vi "initialize_oscilloscope_multiple_waveforms.vi"(0 "Range (0.001 S)":dbl=1.0 format="%#_13g", 1 "error in (no error)":errorcluster) -> (2 "VISA resource name out":refnum<visa-resource-name>, 3 "channels":i32[](array[numeric]), 4 "error out":errorcluster)   [LabVIEW 2016]
doc: "This example shows how to configure multiple channels and acquire waveforms from multiple channels."
uses:
  <instrlib>/Agilent 2000 3000 X-Series/Agilent 2000 3000 X-Series.lvlib
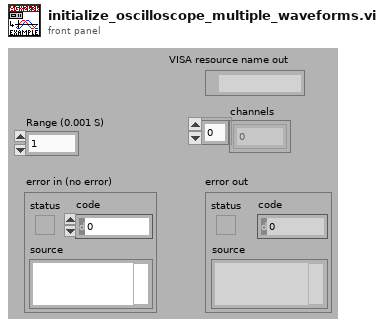
[diagram p1: front panel]
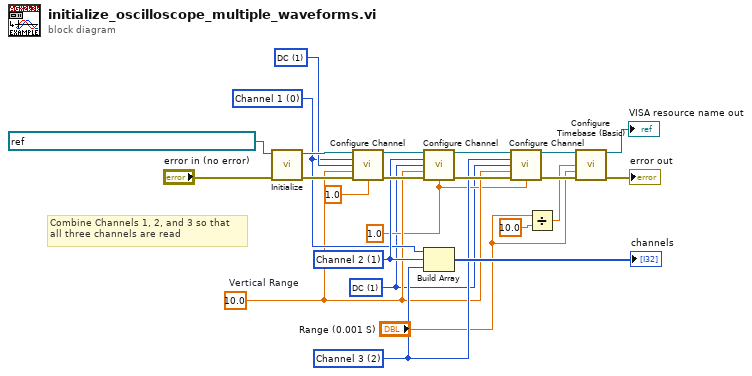
[diagram p0: block diagram]
diagram:
  w8 = 2 items=["Channel 1", "Channel 2", "Channel 3", "Channel 4"] ("Channel Name (0: Channel 1)")
  w6 = 1.0 ("Probe Attenuation (1.0)")
  w5 = 1 items=["AC", "DC", "Ground"] ("Vertical Coupling (1: DC)")
  w17 = 1 items=["AC", "DC", "Ground"] ("Vertical Coupling (1: DC)")
  w14 = 1 items=["Channel 1", "Channel 2", "Channel 3", "Channel 4"] ("Channel (1: Channel 2)")
  w13 = 0 items=["Channel 1", "Channel 2", "Channel 3", "Channel 4"] ("Channel (0: Channel 1)")
  w7 = 10.0  # Vertical Range
  # "Combine Channels 1, 2, and 3 so that\nall three channels are read"
  n1 = call <instrlib>:"Initialize.vi"("error in (no error)"="error in (no error)", "VISA resource name"=refnum<visa-resource-name> "USB0::0x0957::0x1796::MY56272306::INSTR") -> ("error out"=w23:errorcluster, "VISA resource name out"=w22:refnum<visa-resource-name>)  [unwired: 3 in, 5 out]
  n2 = call <instrlib>:"Configure Channel.vi"("VISA resource name"=w22, "Channel Name (0: Channel 1)"=w13, "Coupling (1: DC)"=w17, "Vertical Range (40.0 V)"=w7, "error in (no error)"=w23, "Probe Attenuation (1.0)"=1.0 ("Probe Attenuation (10.0)")) -> ("VISA resource name out"=w21:refnum<visa-resource-name>, "error out"=w20:errorcluster)  [unwired: 5 in, 3 out]
  n3 = call <instrlib>:"Configure Channel.vi"("VISA resource name"=w21, "Channel Name (0: Channel 1)"=w14, "Coupling (1: DC)"=w5, "Vertical Range (40.0 V)"=w7, "error in (no error)"=w20, "Probe Attenuation (1.0)"=w6) -> ("VISA resource name out"=w12:refnum<visa-resource-name>, "error out"=w10:errorcluster)  [unwired: 5 in, 3 out]
  n4 = Build Array(w13, w14, w8) -> (→"channels":i32[])
  n5 = call <instrlib>:"Configure Channel.vi"("VISA resource name"=w12, "Channel Name (0: Channel 1)"=w8, "Coupling (1: DC)"=w5, "Vertical Range (40.0 V)"=w7, "error in (no error)"=w10, "Probe Attenuation (1.0)"=w6) -> ("VISA resource name out"=w11:refnum<visa-resource-name>, "error out"=w9:errorcluster)  [unwired: 5 in, 3 out]
  n6 = Divide(x="Range (0.001 S)", y=10.0) -> (x/y=w2:dbl)
  n7 = call <instrlib>:"Configure Timebase (Basic).vi"("VISA resource name"=w11, "Scale (50 s/div)"=w2, "Range (0.001 S)"="Range (0.001 S)", "error in (no error)"=w9) -> ("VISA resource name out"=→"VISA resource name out":refnum<visa-resource-name>, "error out"=→"error out":errorcluster)  [unwired: 5 in, 5 out]
